vi "tester.vi"() -> ()   [LabVIEW 2024]
uses:
  MyComics.org_class/MyComics.org_class.lvclass/MyComics.org_class.ctl
  MyComics.org_class/MyComics.org_class.lvclass
panel:
  out "series body":string
  out "issue body":string
  out "prev seriesID":i32
  in  "seriesID":i32
  in  "issueID":i32
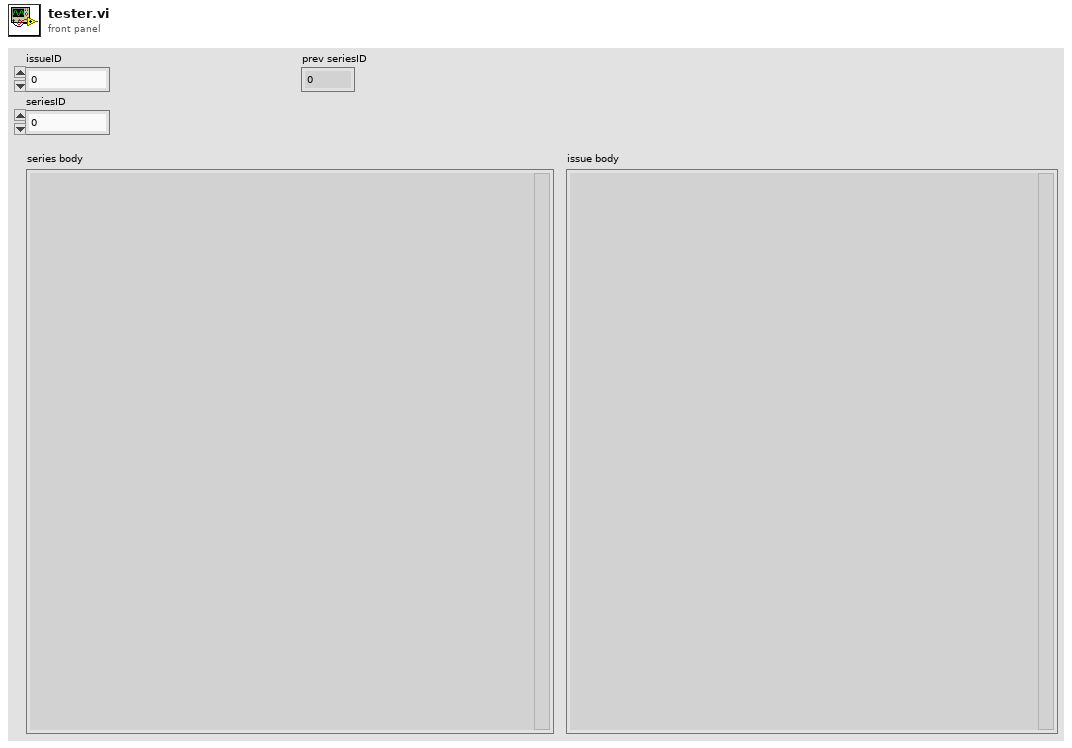
[diagram p1: front panel]
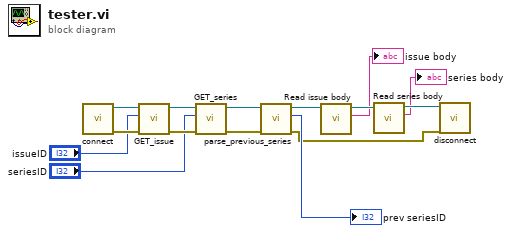
[diagram p0: block diagram]
diagram:
  n1 = call "connect.vi"() -> ("error out"=w14:errorcluster, "MyComics.org_class out"=w15:refnum<class "MyComics.org_class.lvclass">)  [unwired: 10 in]
  n2 = call "GET_issue.vi"("error in (no error)"=w14, "issueID"="issueID", "MyComics.org_class in"=w15) -> ("error out"=w12:errorcluster, "MyComics.org_class out"=w13:refnum<class "MyComics.org_class.lvclass">)  [unwired: 7 in]
  n3 = call "GET_series.vi"("error in (no error)"=w12, "seriesID"="seriesID", "MyComics.org_class in"=w13) -> ("error out"=w8:errorcluster, "MyComics.org_class out"=w9:refnum<class "MyComics.org_class.lvclass">)  [unwired: 7 in]
  n4 = call "parse_previous_series.vi"("error in (no error)"=w8, "MyComics.org_class in"=w9) -> ("error out"=w5:errorcluster, "prev seriesID"=→"prev seriesID":i32, "MyComics.org_class out"=w6:refnum<class "MyComics.org_class.lvclass">)  [unwired: 7 in]
  n5 = call "Read issue body.vi"("MyComics.org_class in"=w6) -> ("issue body"=→"issue body":string, "MyComics.org_class out"=w4:refnum<class "MyComics.org_class.lvclass">)  [unwired: 9 in]
  n6 = call "Read series body.vi"("MyComics.org_class in"=w4) -> ("series body"=→"series body":string, "MyComics.org_class out"=w3:refnum<class "MyComics.org_class.lvclass">)  [unwired: 9 in]
  n7 = call "disconnect.vi"("error in (no error)"=w5, "MyComics.org_class in"=w3) -> ()  [unwired: 8 in, 2 out]
